vi "帮助菜单主VI.vi"() -> ()   [LabVIEW 2014]
doc: "随便选的一个帮助文件"
uses:
  <vilib>/Analysis/NI_AALBase.lvlib
panel:
  in  "停止按钮":bool
  out "波形图表":dbl[](graph)
  # "这是程序前面板截图示意\n\n  截图区域：前面板"
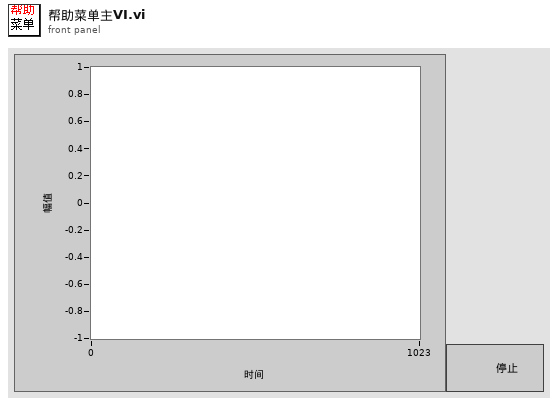
[diagram p1: front panel]
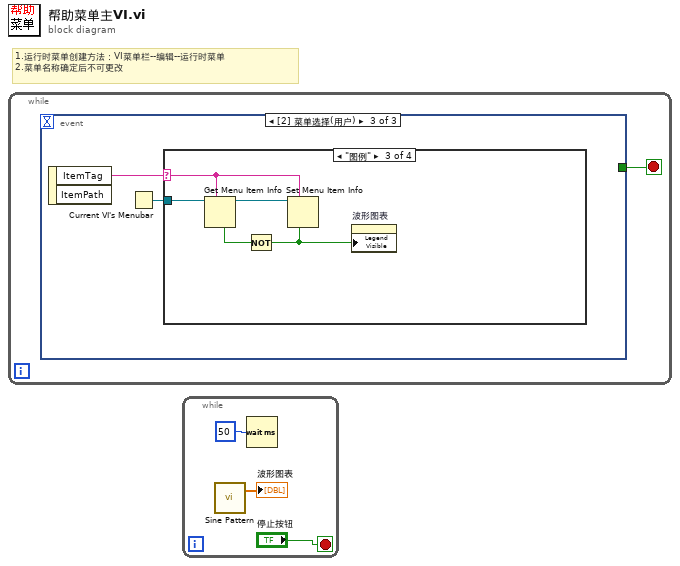
[diagram p0: block diagram]
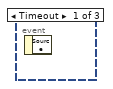
[diagram p2: hidden frame]
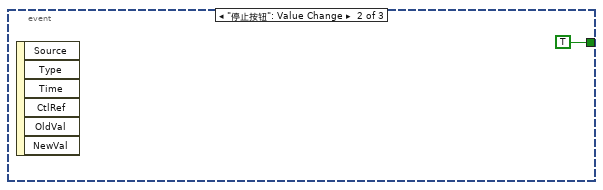
[diagram p3: hidden frame]
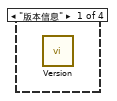
[diagram p4: hidden frame]
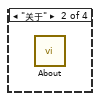
[diagram p5: hidden frame]
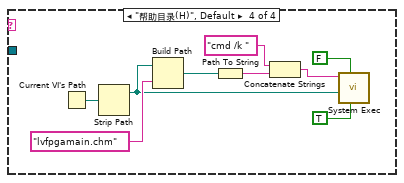
[diagram p6: hidden frame]
diagram:
  # "1.运行时菜单创建方法：VI菜单栏--编辑--运行时菜单\n2.菜单名称确定后不可更改"
  n1 = while {
    stop <- w1 stop-if-true
    n2 = event shown="[2] 菜单选择(用户)" {
      selector: _ -> [_ _ _]
      dyn-events: _ -> [_ _ _]
      timeout: _ -> [_ _ _]
      tunnel: [_ TRUE _] -> w1
      event Timeout {
        n3 = event-data() -> ()  [unwired: 1 in, 1 out]
      }
      event "停止按钮": Value Change {
        n4 = event-data() -> ()  [unwired: 1 in, 6 out]
      }
      event Menu Selection (User) {
        n5 = event-data() -> ("ItemTag"=w4:string)  [unwired: 1 in, 1 out]
        n6 = Current VI's Menubar() -> (w3:refnum<k9>)
        n7 = case shown="\"图例\"" w4 {
          selector: w4 -> [_ _ w6 _]
          tunnel: w3 -> [_ _ w7 _]
          frame "版本信息" {
            n8 = call "Version.vi"() -> ()  [unwired: 12 in]
          }
          frame "关于" {
            n9 = call "About.vi"() -> ()  [unwired: 12 in]
          }
          frame "图例" {
            n10 = Get Menu Item Info(7:w6, 11:w7) -> (3:w8:refnum<k9>, 4:w9:bool)  [unwired: 1 in, 5 out]
            n11 = Not(x=w9) -> (.not. x?=w5:bool)
            n12 = Set Menu Item Info(6:w5, 7:w6, 11:w8) -> ()  [unwired: 4 in, 2 out]
            n13 = property on="波形图表" class="WFChart (严格)"("Legend Visible"=w5) -> ()  [unwired: 2 in, 2 out]
          }
          frame "帮助目录(H)", Default {
            n14 = Current VI's Path() -> (path=w13:path)
            n15 = Strip Path(path=w13) -> (stripped path=w10:path)  [unwired: 1 out]
            n16 = Build Path(base path=w10, name or relative path="lvfpgamain.chm" ("名称或相对路径")) -> (appended path=w11:path)
            n17 = Path To String(path=w11) -> (string=w15:string)
            n18 = Concatenate Strings("cmd /k " ("字符串"), w15) -> (w14:string)
            n19 = call <vilib>:"System Exec.vi"("run minimized? (F)"=TRUE, "wait until completion? (T)"=FALSE, "working directory"=w10, "command line"=w14) -> ()  [unwired: 4 in, 4 out]
          }
        }
      }
    }
  }
  n20 = while {
    stop <- "停止按钮" stop-if-true
    n21 = call <vilib>:"Sine Pattern.vi"() -> ("Sinusoidal Pattern"=→"波形图表":dbl[])  [unwired: 4 in, 1 out]
    n22 = Wait (ms)(milliseconds to wait=u32 50 ("等待时间（毫秒）")) -> ()  [unwired: 1 out]
  }
